vi "testpulseevent.vi"() -> ()   [LabVIEW 2011]
uses:
  kernel32.dll
panel:
  out "数值":i32
  out "返回类型":i32
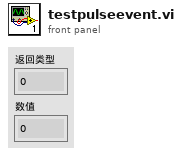
[diagram p1: front panel]
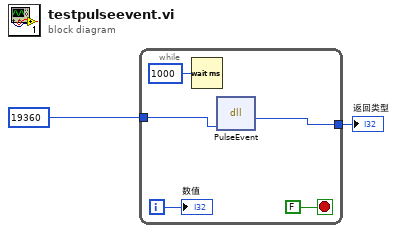
[diagram p0: block diagram]
diagram:
  n1 = while {
    tunnel: u64 19360 ("参数1") -> [w7]
    tunnel: [w6] -> w1
    i -> [w3]
    stop <- FALSE stop-if-true
    n2 = Wait (ms)(milliseconds to wait=u32 1000 ("等待时间（毫秒）")) -> ()  [unwired: 1 out]
    n3 = dll-call lib="kernel32.dll" fn="PulseEvent"("参数1"=w7) -> ("返回类型"=w6:i32)  [unwired: 4 in, 2 out]
    "数值" <- w3
  }
  "返回类型" <- w1
